vi "Centauro Dryer LED Compare.vi"(0 "Actul LED Status":T3={"Damp"=enum."On", "Dry"=enum."Off", "Cool"=enum."Off", "Eco"=enum."Off"}, 1 "Expected LED Status":T3={"Damp"=enum."On", "Dry"=enum."Off", "Cool"=enum."Off", "Eco"=enum."Off"}, 2 "Care":T1, 11 "Error In":errorcluster) -> (4 "Pass/Fail?":bool, 6 "Report Text":string, 15 "Error Out":errorcluster)   [LabVIEW 2016]
uses:
  Centauro Washer/Product Testcode/Centauro/Valew Common/type defs/LED Status OOB.ctl
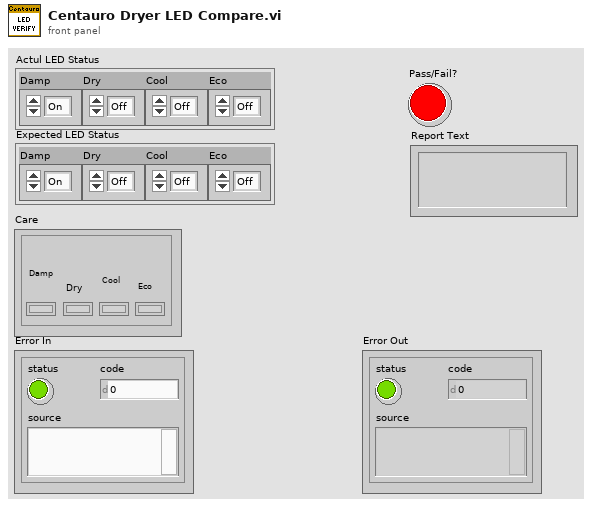
[diagram p1: front panel]
types:
  T1 = cluster{"Damp":bool, "Dry":bool, "Cool":bool, "Eco":bool}
  T2 = typedef "LED Status OOB.ctl" = enum32{"Off", "On", "Blink"}
  T3 = cluster{"Damp":T2, "Dry":T2, "Cool":T2, "Eco":T2}
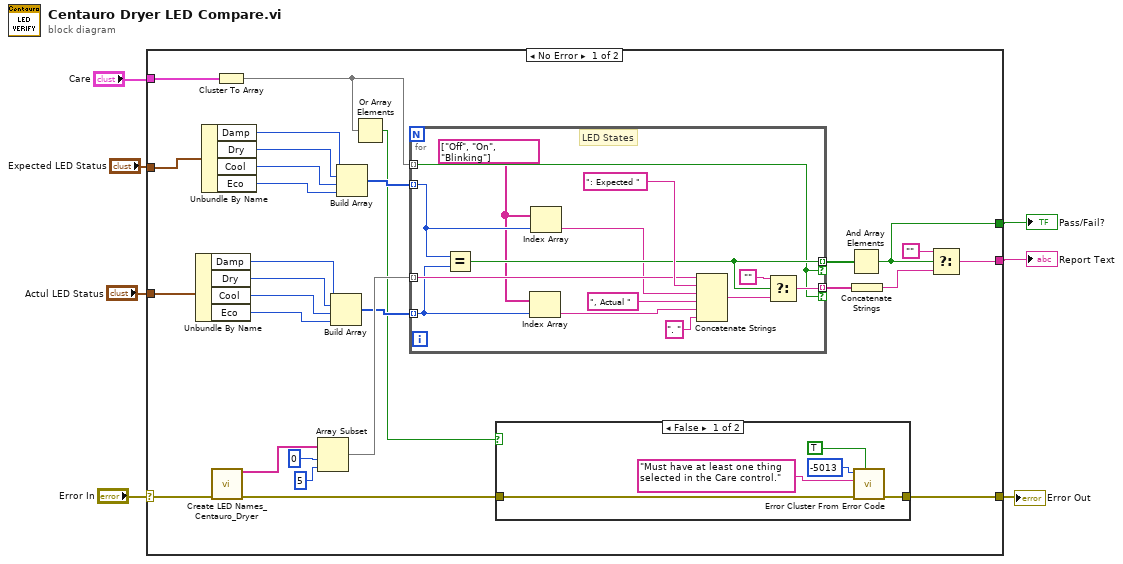
[diagram p0: block diagram]
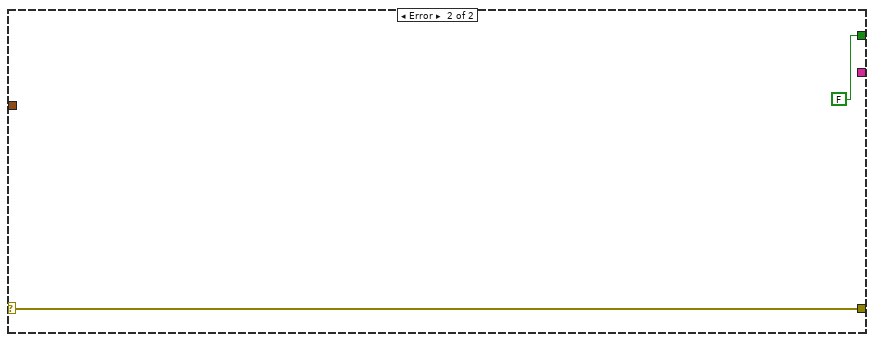
[diagram p3: hidden frame]
diagram:
  n1 = case shown="No Error" "Error In" {
    selector: "Error In" -> [w33 w57]
    tunnel: [w18 w57] -> w1
    tunnel: [w34 _] -> w4
    tunnel: "Care" -> [w32 _]
    tunnel: "Expected LED Status" -> [w16 _]
    tunnel: [w17 FALSE] -> w3
    tunnel: "Actul LED Status" -> [w10 _]
    frame No Error {
      n2 = Unbundle By Name(w10) -> ("Damp"=w12:T2, "Dry"=w13:T2, "Cool"=w14:T2, "Eco"=w15:T2)
      n3 = Unbundle By Name(w16) -> ("Damp"=w22:T2, "Dry"=w21:T2, "Cool"=w20:T2, "Eco"=w19:T2)
      n4 = call "Create LED Names_Centauro_Dryer.vi"("Error In"=w33) -> ("Names"=w26:string[], "Error Out"=w31:errorcluster)  [unwired: 13 in]
      n5 = Cluster To Array(cluster=w32) -> (array=w9:bool[])
      n6 = Array Subset(array=w26, index=0, length=5) -> (w27:string[])
      n7 = Build Array(w12, w13, w14, w15) -> (w11:T2[])
      n8 = Build Array(w22, w21, w20, w19) -> (w30:T2[])
      n9 = Or Array Elements(Boolean array=w9) -> (logical OR=w8:bool)
      n10 = for {
        tunnel: w11 -> [w36] mode=indexing
        tunnel: w30 -> [w39] mode=indexing
        tunnel: [w44] -> w25 mode=indexing if=w42
        tunnel: [w43] -> w23 mode=indexing if=w42
        tunnel: w9 -> [w42] mode=indexing
        tunnel: w27 -> [w41] mode=indexing
        w37 = string[] ["Off", "On", "Blinking"]
        # "LED States"
        n11 = Equal?(x=w39, y=w36) -> (x = y?=w43:bool)
        n12 = Index Array(array=w37, index=w36) -> (element=w38:string)
        n13 = Index Array(array=w37, index=w39) -> (element=w40:string)
        n14 = Concatenate Strings(w41, ": Expected " ("string"), w40, ", Actual " ("string"), w38, ". " ("string")) -> (w45:string)
        n15 = Select(t="", s=w43, f=w45) -> (s? t:f=w44:string)
      }
      n16 = case shown="False" w8 {
        tunnel: w31 -> [w54 w55]
        tunnel: [w53 w55] -> w18
        frame False {
          n17 = call <vilib>:"Error Cluster From Error Code.vi"("show call chain? (False)"=TRUE, "error in (no error)"=w54, "error message (\"\")"="Must have at least one thing selected in the Care control." ("error message (\"\")"), "error code (0)"=-5013) -> ("error out"=w53:errorcluster)  [unwired: 5 in]
        }
        frame True {
        }
      }
      n18 = And Array Elements(Boolean array=w23) -> (logical AND=w17:bool)
      n19 = Concatenate Strings(w25) -> (w24:string)
      n20 = Select(t="", s=w17, f=w24) -> (s? t:f=w34:string)
    }
    frame Error {
    }
  }
  "Report Text" <- w4
  "Pass/Fail?" <- w3
  "Error Out" <- w1
